vi "Calculation of SMD-2016.vi"() -> ()   [LabVIEW 2016]
panel:
  out "坐标":dbl
  out "高度":dbl
  out "宽度":dbl
  in  "高":dbl
  in  "总宽":dbl
  in  "间距":dbl
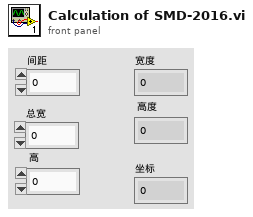
[diagram p1: front panel]
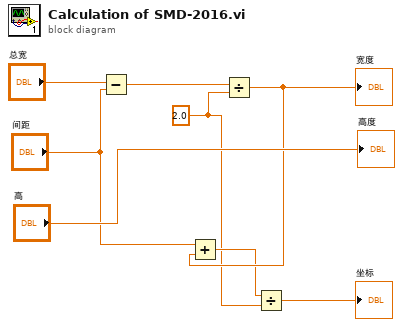
[diagram p0: block diagram]
diagram:
  w2 = 2.0 ("y")
  n1 = Subtract(x="总宽", y="间距") -> (x-y=w7:dbl)
  n2 = Divide(x=w7, y=w2) -> (x/y=w4:dbl)
  "宽度" <- w4
  n3 = Add(x="间距", y=w4) -> (x+y=w3:dbl)
  n4 = Divide(x=w3, y=w2) -> (x/y=→"坐标":dbl)
  "高度" <- "高"
